vi "Custom Assertion Failure Message.vi"() -> (0 "error out":errorcluster)   [LabVIEW 2017, in "Assertion.Tests.lvlib" / "Assert String Not Contains String Ignoring Case.lvlib"]
uses:
  Assert String Not Contains String Ignoring Case.lvlib
  Assertion/Assertion.lvlib
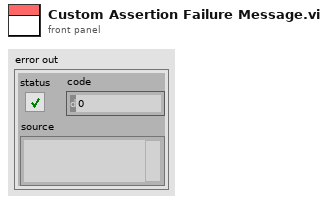
[diagram p1: front panel]
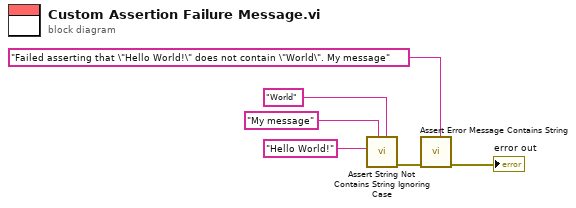
[diagram p0: block diagram]
diagram:
  n1 = call "Assert String Not Contains String Ignoring Case.vi"("Needle"="World", "Message (\"\")"="My message" ("Message (\"\")"), "Haystack"="Hello World!") -> ("error out"=w2:errorcluster)  [unwired: 8 in]
  n2 = call "Assert Error Message Contains String.vi"("Expected"="Failed asserting that \"Hello World!\" does not contain \"World\". My message", "error in (no error)"=w2) -> ("error out"=→"error out":errorcluster)  [unwired: 9 in]
